vi "Simultaneous_2_Edge_Sep_example.vi"() -> ()   [LabVIEW 2014]
doc: "I. Description:\nThis example demonstrates how to perform a finite number of two edge separation measurements on a Counter Input Channel. The First Edge, Second Edge, Minimum Value, Maximum Value, and Samples to Read are all configurable. \n\nThis example shows how to perform a two edge separation measurement on the counter's default input terminals (refer to section IV, I/O Connections Overview, below for more information), but could easily be expanded to measure two edge separation on any PFI, RTSI, or internal signal.\n\nRefer to your device documentation to see if your device supports two edge separation measurements.\n\nII. Instructions for Running:\n1. Select the Physical Channel which corresponds to the counter on the DAQ device you want to perform a two edge separation measurement on.\n2. Enter the First Edge and Second Edge corresponding to the two edges you want the counter to measure. Enter the Maximum and Minimum Value to specify the range of your unknown two edge separation. Additionally, you can change the First and Second Edge Input Terminals using the channel property node.\nNote: It is important to set the Maximum and Minimum Values of your unknown two edge separation as accurately as possible so the best internal timebase can be chosen to minimize measurement error. The default values specify a range that can be measured by the counter using the 20MHzTimebase.\n3. Set the Samples to Read control. This will determine how many samples are read each time the while loop iterates.\n\nIII. Block Diagram Steps:\n1. Create a Counter Input channel to perform a Two Edge Separation measurement. The First and Second Edge parameters are used to specify the rising or falling edge of one digital signal and the rising or falling edge of another digital signal. It is important to set the Maximum and Minimum Values of your unknown two edge separation as accurately as possible so the best internal timebase can be chosen to minimize measurement error. The default values specify a range that can be measured by the counter using the 20MHzTimebase.\n2. Call the DAQmx Timing VI (Implicit) to configure the Sample Mode and Samples per Channel. Note: For time measurements with counters, the implicit timing VI is used because the signals being measured determine the sample rate. \n3. Call the Start VI to arm the counter and begin measuring.\n4. For finite measurements, the counter will stop reading data when the Samples per Channel have been received. \n5. Call the Clear Task VI to clear the Task.\n6. Use the popup dialog box to display an error if any.\n\nIV. I/O Connections Overview:\nThe counter will perform a two edge separation measurement on the First and Second Edge Input Terminals of the counter specified in the Physical Channel I/O control. \n\n In this example the two edge separation will be measured on the default input terminals on ctr0. \n\nFor more information on the default counter input and output terminals for your device, open the NI-DAQmx Help, and refer to Counter Signal Connections found under the Device Considerations book in the table of contents."
uses:
  <vilib>/Utility/error.llb/DialogType.ctl
  <vilib>/DAQmx/read.llb/DAQmx Read (Counter DBL 1Chan 1Samp).vi
  <vilib>/DAQmx/configure/timing.llb/DAQmx Timing (Implicit).vi
  <vilib>/DAQmx/create/channels.llb/DAQmx Create Channel (CI-Two Edge Separation).vi
panel:
  out "armed":bool
  in  "ARM":bool
  in  "stop":bool
  in  "Counter 2":tag="LightScreens/ctr1"
  out "Data 1 (sec)":dbl caption="Waveform" format="%0.9f"
  out "Data 0 (sec)":dbl caption="Waveform" format="%0.9f"
  in  "Second Edge":i32(ring)=10280 items=["Rising"=10280, "Falling"=10171]
  in  "First Edge":i32(ring)=10280 items=["Rising"=10280, "Falling"=10171]
  in  "Counter 1":tag="LightScreens/ctr0"
  in  "Min Value (sec)":dbl=1e-05 caption="Minimum Value (sec)" format="%0.9f"
  in  "Max Value (sec)":dbl=0.005 caption="Maximum Value (sec)" format="%0.9f"
  in  "Samples per Chnl":i32=1 caption="Samples per Channel"
  # "Channel Parameters"
  # "Timing Parameters"
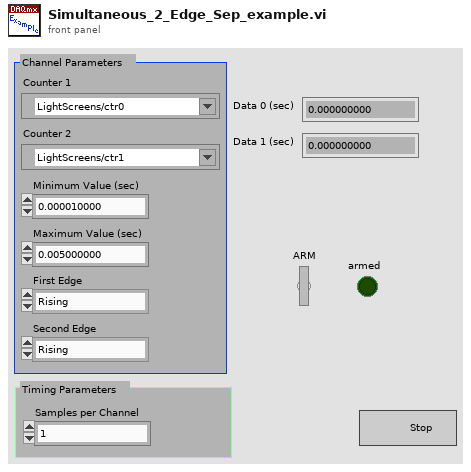
[diagram p1: front panel]
types:
  T1 = typedef "DialogType.ctl" = u16
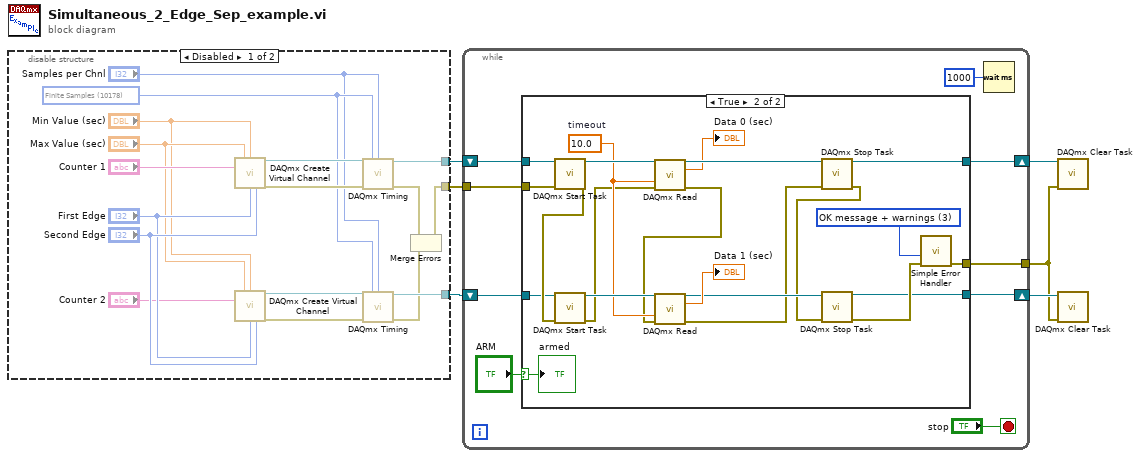
[diagram p0: block diagram]
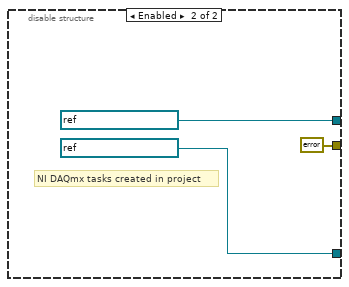
[diagram p2: hidden frame]
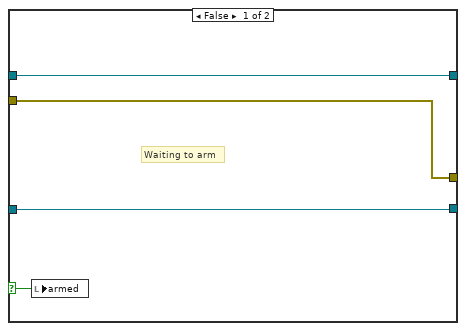
[diagram p3: hidden frame]
diagram:
  n1 = disable-structure shown="Disabled" {
    disable-tunnel: [w7 errorcluster {"status"=FALSE, "code"=0, "source"=""} ("error in")] -> w4
    disable-tunnel: [w23 refnum<k21> "TwoEdgeSepCtr0" ("task/channels in")] -> w6
    disable-tunnel: [w17 refnum<k21> "TwoEdgeSepCtr1" ("task/channels in")] -> w5
    frame Disabled {
      w11 = 10178 items=["Finite Samples"=10178, "Continuous Samples"=10123] ("sample mode")
      n2 = call-poly <vilib>:"DAQmx Create Virtual Channel.vi"("maximum value"="Max Value (sec)", "minimum value"="Min Value (sec)", "counter"="Counter 1", "first edge"="First Edge", "second edge"="Second Edge") -> ("task out"=w21:refnum<k21>, "error out"=w22:errorcluster)  [unwired: 9 in]
      n3 = call-poly <vilib>:"DAQmx Create Virtual Channel.vi"("maximum value"="Max Value (sec)", "minimum value"="Min Value (sec)", "counter"="Counter 2", "first edge"="First Edge", "second edge"="Second Edge") -> ("task out"=w19:refnum<k21>, "error out"=w18:errorcluster)  [unwired: 9 in]
      n4 = call-poly <vilib>:"DAQmx Timing.vi"("task/channels in"=w21, "sample mode"=w11, "samples per channel"="Samples per Chnl", "error in"=w22) -> ("task out"=w23:refnum<k21>, "error out"=w9:errorcluster)  [unwired: 10 in]
      n5 = call-poly <vilib>:"DAQmx Timing.vi"("task/channels in"=w19, "sample mode"=w11, "samples per channel"="Samples per Chnl", "error in"=w18) -> ("task out"=w17:refnum<k21>, "error out"=w8:errorcluster)  [unwired: 10 in]
      n6 = Merge Errors(w9, w8) -> (w7:errorcluster)
    }
    frame Enabled {
      # "NI DAQmx tasks created in project"
    }
  }
  n7 = while {
    shift-right: [w34] -> w2
    shift-left: w6 -> [w31]
    shift-right: [w32] -> w3
    shift-left: w5 -> [w30]
    tunnel: w4 -> [w29]
    tunnel: [w28] -> w1
    stop <- "stop" stop-if-true
    n8 = case shown="True" "ARM" {
      selector: "ARM" -> [w36 w40]
      tunnel: [w39 w46] -> w34
      tunnel: [w38 w45] -> w32
      tunnel: w31 -> [w39 w44]
      tunnel: w30 -> [w38 w43]
      tunnel: w29 -> [w37 w42]
      tunnel: [w37 w41] -> w28
      frame False {
        # "Waiting to arm"
        n9 = local write "armed"(w36) -> ()
      }
      frame True {
        w53 = 10.0  # timeout
        w54 = T1 3 items=["no dialog", "OK message", "continue or stop message", "OK message + warnings", "continue/stop + warnings"] ("type of dialog (OK msg:1)")
        n10 = call <vilib>:"DAQmx Start Task.vi"("task/channels in"=w44, "error in"=w42) -> ("task out"=w60:refnum<k21>, "error out"=w52:errorcluster)  [unwired: 12 in]
        n11 = call <vilib>:"DAQmx Start Task.vi"("task/channels in"=w43, "error in"=w52) -> ("task out"=w55:refnum<k21>, "error out"=w51:errorcluster)  [unwired: 12 in]
        n12 = call-poly <vilib>:"DAQmx Read.vi"("task/channels in"=w60, "timeout"=w53, "error in"=w51) -> ("task out"=w59:refnum<k21>, "data"=→"Data 0 (sec)":dbl, "error out"=w50:errorcluster)  [unwired: 10 in]
        n13 = call-poly <vilib>:"DAQmx Read.vi"("task/channels in"=w55, "timeout"=w53, "error in"=w50) -> ("task out"=w56:refnum<k21>, "data"=→"Data 1 (sec)":dbl, "error out"=w49:errorcluster)  [unwired: 10 in]
        n14 = call <vilib>:"DAQmx Stop Task.vi"("task/channels in"=w59, "error in"=w49) -> ("task out"=w46:refnum<k21>, "error out"=w48:errorcluster)  [unwired: 12 in]
        n15 = call <vilib>:"DAQmx Stop Task.vi"("task/channels in"=w56, "error in"=w48) -> ("task out"=w45:refnum<k21>, "error out"=w47:errorcluster)  [unwired: 12 in]
        n16 = call <vilib>:"Simple Error Handler.vi"("type of dialog (OK msg:1)"=w54, "error in (no error)"=w47) -> ("error out"=w41:errorcluster)  [unwired: 3 in, 4 out]
        "armed" <- w40
      }
    }
    n17 = Wait (ms)(milliseconds to wait=u32 1000) -> ()  [unwired: 1 out]
  }
  n18 = call <vilib>:"DAQmx Clear Task.vi"("task in"=w2, "error in"=w1) -> ()  [unwired: 13 in, 1 out]
  n19 = call <vilib>:"DAQmx Clear Task.vi"("task in"=w3, "error in"=w1) -> ()  [unwired: 13 in, 1 out]
